vi "GetRangeAndUnits.vi"(0 "Handle":u32, 1 "Controller Channel":i32) -> (7 "FT_Status":u32(ring) items=["FT_OK", "FT_INVALID_HANDLE", "FT_DEVICE_NOT_FOUND", "FT_DEVICE_NOT_OPENED", "FT_IO_ERROR", "FT_INSUFFICIENT_RESOURCES", "FT_INVALID_PARAMETER", "FT_INVALID_BAUD_RATE", "FT_DEVICE_NOT_OPENED_FOR_ERASE", "FT_DEVICE_NOT_OPENED_FOR_WRITE", "FT_FAILED_TO_WRITE_DEVICE", "FT_EEPROM_READ_FAILED", "FT_EEPROM_WRITE_FAILED", "FT_EEPROM_ERASE_FAILED", "FT_EEPROM_NOT_PRESENT", "FT_EEPROM_NOT_PROGRAMMED", "FT_INVALID_ARGS", "FT_NOT_SUPPORTED", "FT_OTHER_ERROR"], 9 "Range":i32, 10 "Range Units":string)   [LabVIEW 2013]
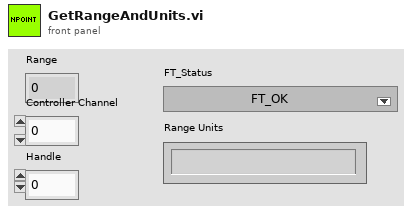
[diagram p1: front panel]
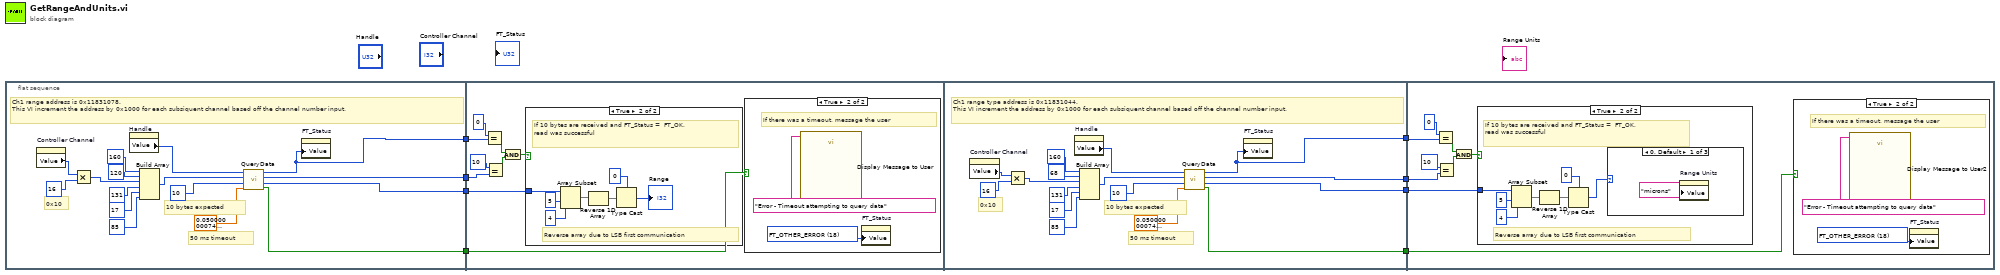
[diagram p0: block diagram]
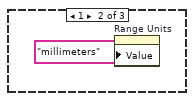
[diagram p6: hidden frame]
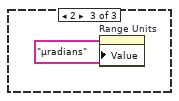
[diagram p7: hidden frame]
diagram:
  n1 = flat-sequence {
    tunnel: [w15] -> w8
    tunnel: [w14] -> w7
    tunnel: [w13] -> w6
    tunnel: [w12] -> w5
    tunnel: w8 -> [w33]
    tunnel: w7 -> [w31]
    tunnel: w6 -> [w30]
    tunnel: w5 -> [w28]
    tunnel: [w45] -> w4
    tunnel: [w49] -> w3
    tunnel: [w48] -> w2
    tunnel: [w47] -> w1
    tunnel: w4 -> [w62]
    tunnel: w3 -> [w59]
    tunnel: w2 -> [w61]
    tunnel: w1 -> [w60]
    frame #0 {
      # "10 bytes expected"
      # "50 ms timeout"
      # "Ch1 range address is 0x11831078.\nThis VI increment the address by 0x1000 for each subsiquent channel based off the channel number input."
      # "0x10"
      n2 = property on="Controller Channel" class="DigNum (strict)"() -> ("Value"=w10:i32)  [unwired: 2 in, 2 out]
      n3 = Multiply(x=w10, y=u8 16) -> (x*y=w11:i32)
      n4 = property on="Handle" class="DigNum (strict)"() -> ("Value"=w9:u32)  [unwired: 2 in, 2 out]
      n5 = Build Array(u8 160 ("element"), u8 120 ("element"), w11, u8 131 ("element"), u8 17 ("element"), u8 85 ("element")) -> (w18:i32[])
      n6 = call "QueryData.vi"("TimeoutLengthSeconds"=sgl 0.05, "NumBytesExpected"=u32 10, "Message"=w18, "Handle"=w9) -> ("Timeout"=w13:bool, "Return Array"=w14:u8[], "Bytes Read"=w15:u32, "FT_Status"=w12:u32)  [unwired: 4 in]
      n7 = property on="FT_Status" class="Ring (strict)"("Value"=w12) -> ()  [unwired: 2 in, 2 out]
    }
    frame #1 {
      n8 = Equal?(x=u32 0, y=w28) -> (x = y?=w26:bool)
      n9 = Equal?(x=u32 10, y=w33) -> (x = y?=w27:bool)
      n10 = And(x=w26, y=w27) -> (x .and. y?=w25:bool)
      n11 = case shown="True" w25 {
        tunnel: w31 -> [_ w42]
        frame False {
        }
        frame True {
          # "Reverse array due to LSB first communication"
          # "If 10 bytes are received and FT_Status =  FT_OK,\nread was successful"
          n12 = Array Subset(array=w42, index=5, length=4) -> (w38:u8[])
          n13 = Reverse 1D Array(array=w38) -> (reversed array=w37:u8[])
          n14 = Type Cast(type=0, x=w37) -> (*(type *) &x=→"Range":i32)
        }
      }
      n15 = case shown="True" w30 {
        frame False {
        }
        frame True {
          w34 = u32 18 items=["FT_OK", "FT_INVALID_HANDLE", "FT_DEVICE_NOT_FOUND", "FT_DEVICE_NOT_OPENED", "FT_IO_ERROR", "FT_INSUFFICIENT_RESOURCES", "FT_INVALID_PARAMETER", "FT_INVALID_BAUD_RATE", "FT_DEVICE_NOT_OPENED_FOR_ERASE", "FT_DEVICE_NOT_OPENED_FOR_WRITE", "FT_FAILED_TO_WRITE_DEVICE", "FT_EEPROM_READ_FAILED", "FT_EEPROM_WRITE_FAILED", "FT_EEPROM_ERASE_FAILED", "FT_EEPROM_NOT_PRESENT", "FT_EEPROM_NOT_PROGRAMMED", "FT_INVALID_ARGS", "FT_NOT_SUPPORTED", "FT_OTHER_ERROR"] ("FT_Status")
          # "If there was a timeout, message the user"
          n16 = call "Display Message to User"("Message"="Error - Timeout attempting to query data") -> ()  [unwired: 9 in, 2 out]
          n17 = property on="FT_Status" class="Ring (strict)"("Value"=w34) -> ()  [unwired: 2 in, 2 out]
        }
      }
    }
    frame #2 {
      # "10 bytes expected"
      # "50 ms timeout"
      # "Ch1 range type address is 0x11831044.\nThis VI increment the address by 0x1000 for each subsiquent channel based off the channel number input."
      # "0x10"
      n18 = property on="Controller Channel" class="DigNum (strict)"() -> ("Value"=w44:i32)  [unwired: 2 in, 2 out]
      n19 = Multiply(x=w44, y=u8 16) -> (x*y=w46:i32)
      n20 = property on="Handle" class="DigNum (strict)"() -> ("Value"=w43:u32)  [unwired: 2 in, 2 out]
      n21 = Build Array(u8 160 ("element"), u8 68 ("element"), w46, u8 131 ("element"), u8 17 ("element"), u8 85 ("element")) -> (w52:i32[])
      n22 = call "QueryData.vi"("TimeoutLengthSeconds"=sgl 0.05, "NumBytesExpected"=u32 10, "Message"=w52, "Handle"=w43) -> ("Timeout"=w47:bool, "Return Array"=w48:u8[], "Bytes Read"=w49:u32, "FT_Status"=w45:u32)  [unwired: 4 in]
      n23 = property on="FT_Status" class="Ring (strict)"("Value"=w45) -> ()  [unwired: 2 in, 2 out]
    }
    frame #3 {
      n24 = Equal?(x=u32 0, y=w62) -> (x = y?=w64:bool)
      n25 = Equal?(x=u32 10, y=w59) -> (x = y?=w65:bool)
      n26 = And(x=w64, y=w65) -> (x .and. y?=w63:bool)
      n27 = case shown="True" w63 {
        tunnel: w61 -> [_ w76]
        frame False {
        }
        frame True {
          # "Reverse array due to LSB first communication"
          # "If 10 bytes are received and FT_Status =  FT_OK,\nread was successful"
          n28 = Array Subset(array=w76, index=5, length=4) -> (w72:u8[])
          n29 = Reverse 1D Array(array=w72) -> (reversed array=w71:u8[])
          n30 = Type Cast(type=0, x=w71) -> (*(type *) &x=w70:i32)
          n31 = case shown="0, Default" w70 {
            frame 0, Default {
              n32 = property on="Range Units" class="Str"("Value"="microns" ("Range Units")) -> ()  [unwired: 2 in, 2 out]
            }
            frame 1 {
              n33 = property on="Range Units" class="Str"("Value"="millimeters" ("Range Units")) -> ()  [unwired: 2 in, 2 out]
            }
            frame 2 {
              n34 = property on="Range Units" class="Str"("Value"="µradians" ("Range Units")) -> ()  [unwired: 2 in, 2 out]
            }
          }
        }
      }
      n35 = case shown="True" w60 {
        frame False {
        }
        frame True {
          w68 = u32 18 items=["FT_OK", "FT_INVALID_HANDLE", "FT_DEVICE_NOT_FOUND", "FT_DEVICE_NOT_OPENED", "FT_IO_ERROR", "FT_INSUFFICIENT_RESOURCES", "FT_INVALID_PARAMETER", "FT_INVALID_BAUD_RATE", "FT_DEVICE_NOT_OPENED_FOR_ERASE", "FT_DEVICE_NOT_OPENED_FOR_WRITE", "FT_FAILED_TO_WRITE_DEVICE", "FT_EEPROM_READ_FAILED", "FT_EEPROM_WRITE_FAILED", "FT_EEPROM_ERASE_FAILED", "FT_EEPROM_NOT_PRESENT", "FT_EEPROM_NOT_PROGRAMMED", "FT_INVALID_ARGS", "FT_NOT_SUPPORTED", "FT_OTHER_ERROR"] ("FT_Status")
          # "If there was a timeout, message the user"
          n36 = call "Display Message to User2"("Message"="Error - Timeout attempting to query data") -> ()  [unwired: 9 in, 2 out]
          n37 = property on="FT_Status" class="Ring (strict)"("Value"=w68) -> ()  [unwired: 2 in, 2 out]
        }
      }
    }
  }
